vi "Create All Message Queues.vi"(8 "error in (no error)":errorcluster) -> (0 "error out":errorcluster, 2 "Queues Array":refnum<queue>[](array[refnum]), 3 "Message Queues out":T1)   [LabVIEW 2019, in "Message Queue.lvlib"]
doc: "This VI creates and initializes all the message queues for your application. If your application requires more than one message queue, right-click the \"Message Queues\" constant above and select Open Type Def. Add the new Message Queue(s) to the type definition, then initialize them in this VI."
uses:
  Message Queue.lvlib
  All Message Queues.ctl
  Message Cluster.ctl
  Enqueue Message (Single).vi
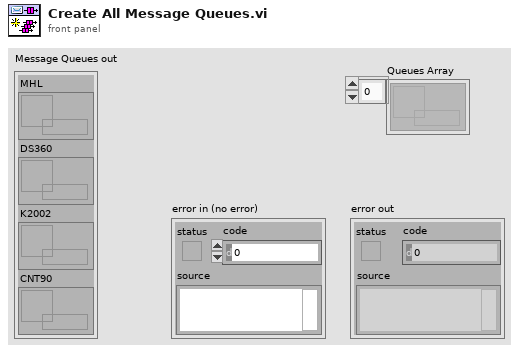
[diagram p1: front panel]
types:
  T1 = typedef "Message Queue.lvlib/All Message Queues.ctl" = cluster{"MHL":refnum<queue>, "DS360":refnum<queue>, "K2002":refnum<queue>, "CNT90":refnum<queue>}
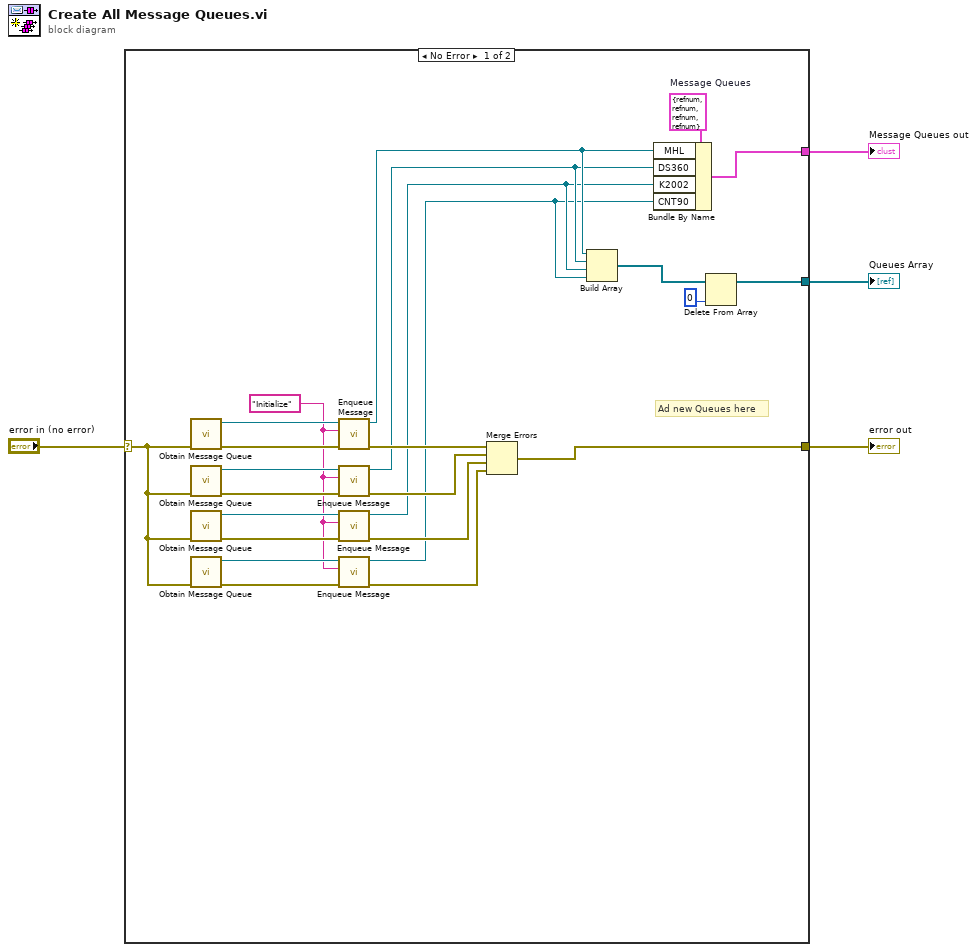
[diagram p0: block diagram]
diagram:
  n1 = case shown="No Error" "error in (no error)" {
    selector: "error in (no error)" -> [w12 w29]
    tunnel: [w16 w29] -> w4
    tunnel: [w26 _] -> w3
    tunnel: [w5 _] -> w1
    frame No Error {
      w17 = "Initialize" ("Message")
      w27 = T1 {"MHL"=refnum, "DS360"=refnum, "K2002"=refnum, "CNT90"=refnum}  # Message Queues
      # "Ad new Queues here"
      n2 = call "Obtain Message Queue.vi"("error in (no error)"=w12) -> ("error out"=w25:errorcluster, "Message Queue"=w24:refnum<queue>)  [unwired: 9 in]
      n3 = call "Obtain Message Queue.vi"("error in (no error)"=w12) -> ("error out"=w22:errorcluster, "Message Queue"=w23:refnum<queue>)  [unwired: 9 in]
      n4 = call "Obtain Message Queue.vi"("error in (no error)"=w12) -> ("error out"=w21:errorcluster, "Message Queue"=w20:refnum<queue>)  [unwired: 9 in]
      n5 = call "Obtain Message Queue.vi"("error in (no error)"=w12) -> ("error out"=w18:errorcluster, "Message Queue"=w19:refnum<queue>)  [unwired: 9 in]
      n6 = call-poly "Enqueue Message.vi"("error in (no error)"=w25, "Message"=w17, "Message Queue"=w24) -> ("error out"=w28:errorcluster, "dup Message Queue"=w9:refnum<queue>)  [unwired: 7 in]
      n7 = call-poly "Enqueue Message.vi"("error in (no error)"=w22, "Message"=w17, "Message Queue"=w23) -> ("error out"=w15:errorcluster, "dup Message Queue"=w8:refnum<queue>)  [unwired: 7 in]
      n8 = call-poly "Enqueue Message.vi"("error in (no error)"=w21, "Message"=w17, "Message Queue"=w20) -> ("error out"=w14:errorcluster, "dup Message Queue"=w7:refnum<queue>)  [unwired: 7 in]
      n9 = call-poly "Enqueue Message.vi"("error in (no error)"=w18, "Message"=w17, "Message Queue"=w19) -> ("error out"=w13:errorcluster, "dup Message Queue"=w6:refnum<queue>)  [unwired: 7 in]
      n10 = Merge Errors(w28, w15, w14, w13) -> (w16:errorcluster)
      n11 = Build Array(w9, w8, w7, w6) -> (w11:refnum<queue>[])
      n12 = Bundle By Name(cluster=w27, "MHL"=w9, "DS360"=w8, "K2002"=w7, "CNT90"=w6) -> (w26:T1)
      n13 = Delete From Array(array=w11, index=0) -> (array with subset deleted=w5:refnum<queue>[])  [unwired: 1 in, 1 out]
    }
    frame Error {
    }
  }
  "Message Queues out" <- w3
  "error out" <- w4
  "Queues Array" <- w1
